vi "oldVisionToGame.vi"(4 "VSS_Ref":T1={"FoulQuadrantVSS"=enum."NO_QUADRANT", "TeamColorVSS"=enum."YELLOW", "HalfVSS"=enum."NO_HALF", "Foul"=enum."FREE_KICK", "timestamp"=0.0}, 5 "Defense stretch":i32=500, 6 "Team/ Side":u16[](array[numeric]), 7 "Defense width":i32=1000, 8 "error in (no error)":errorcluster, 9 "touch":bool, 10 "IA State":T2={"our_robots"=[], "enemy_robots"=[], "balls"=[], "geometry"={"line_width"=0, "field_length"=0, "field_width"=0, "boundary_width"=0, "referee_width"=0, "goal_width"=0, "goal_depth"=0, "goal_wall_width"=0, "center_circle_radius"=0, "defense_radius"=0, "defense_stretch"=0, "free_kick_from_defense_dist"=0, "penalty_spot_from_field_line_dist"=0, "penalty_line_from_spot_dist"=0}, "IA Judge"={"stage"="", "command"="", "our_goalie_id"=0.0, "enemy_goalie_id"=0.0, "command enum"=enum."Halt", "Time"=enum."Azul"}, "Received Timestamp"=timestamp(0 s since 1904-01-01), "Events"={"Touch"=FALSE, "Ball out"=FALSE, "id touch"=0.0, "Ball out of \nVision"=FALSE, "Ball inside \nGoalie area"=FALSE, "Robot not responding"=FALSE, "Robots responding status"=[1.0, 1.0, 1.0, 1.0, 1.0, 1.0], "Enemy Ball \nPossession"=FALSE, "Pass State"=FALSE, "id end of pass"=0.0, "Kick"=FALSE, "Id ini Possession"=0.0, "Ball Possesion"=FALSE, "Id Possesion"=0.0, "Direct Kick"=FALSE, "2nd Strk Ativo"=FALSE}}, 11 "Game in":refnum<class "Game.lvclass">) -> (0 "error out":errorcluster, 3 "Game out":refnum<class "Game.lvclass">)   [LabVIEW 2023, in "Game.lvclass"]
uses:
  Game.lvclass
  Vision_class/Old vision/SSL Detection Frame Simple Estimator Cameras VelCmd Folder/Core/AI Input.ctl
  Vision_class/Old vision/Controls/AI Robot.ctl
  Vision_class/Old vision/Controls/Functions Enum.ctl
  Vision_class/Old vision/Controls/AttackerStates.ctl
  Vision_class/Old vision/Controls/PathDests.ctl
  Vision_class/Old vision/Controls/PathDest.ctl
  Navigation/VSSNavigation/VSSAttackerStates.ctl
  Vision_class/Old vision/SSL Detection Frame Simple Estimator Cameras VelCmd Folder/Core/AI Ball.ctl
  Vision_class/Old vision/SSL Detection Frame Simple Estimator Cameras VelCmd Folder/Core/Field Size.ctl
  Vision_class/Old vision/SSL Detection Frame Simple Estimator Cameras VelCmd Folder/Core/AI Judge.ctl
  Communication_class/Paths/MessageAI_State Folder/Intel/Command Enum.ctl
  Vision_class/Old vision/SSL Detection Frame Simple Estimator Cameras VelCmd Folder/Util/Events/Events.ctl
  Referee_class/VSS_Ref.ctl
  Game.lvclass/Game.ctl
  Write FieldRef.vi
  Write AllyRef.vi
  Write EnemyRef.vi
  Write BallRef.vi
  Write TimeRef.vi
  Write Referee.vi
  Read FieldRef.vi
  Read AllyRef.vi
  Read EnemyRef.vi
  Read BallRef.vi
  Read Referee.vi
  Field_class/Field.lvclass
  Ally_class/Ally.lvclass
  Enemy_class/Enemy.lvclass
  Ball_class/Ball.lvclass
  Referee_class/Referee.lvclass
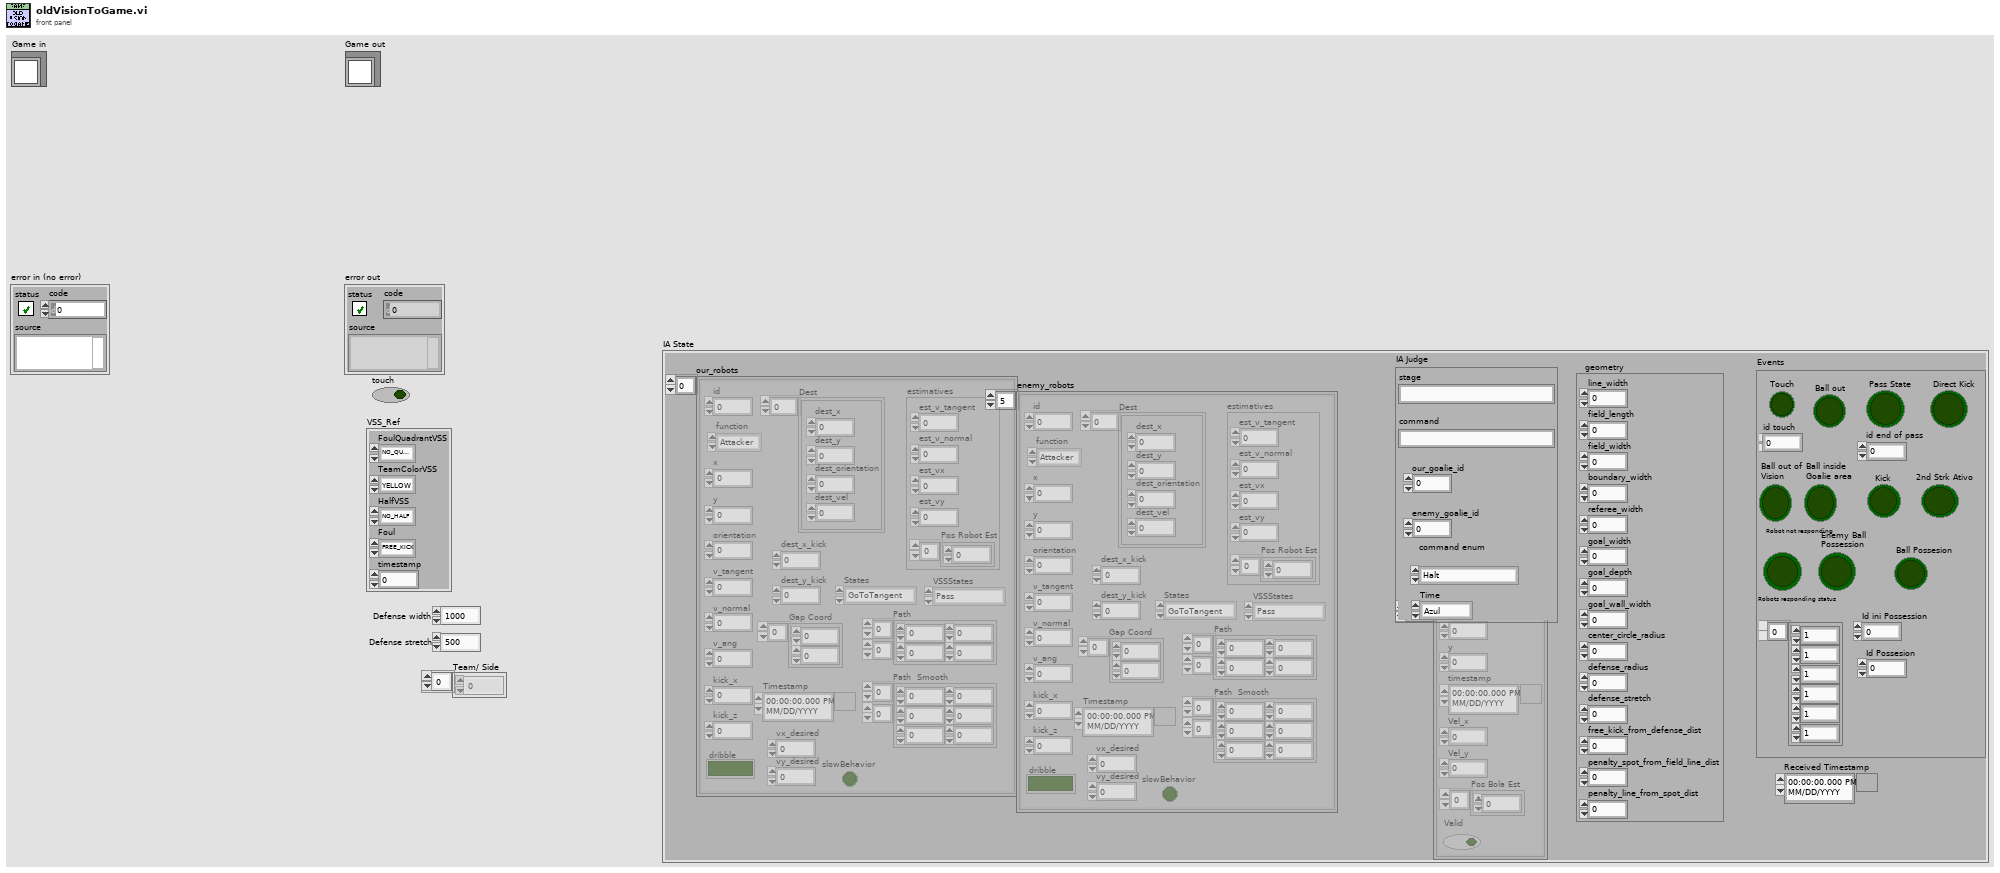
[diagram p1: front panel]
types:
  T1 = typedef "VSS_Ref.ctl" = cluster{"FoulQuadrantVSS":enum16{"NO_QUADRANT", "QUADRANT_1", "QUADRANT_2", "QUADRANT_3", "QUADRANT_4"}, "TeamColorVSS":enum16{"BLUE", "YELLOW", "NONE"}, "HalfVSS":enum16{"NO_HALF", "FIRST_HALF", "SECOND_HALF", "OVERTIME_FIRST_HALF", "OVERTIME_SECOND_HALF", "PENALTY_SHOOTOUS"}, "Foul":enum16{"FREE_KICK", "PENALTY_KICK", "GOAL_KICK", "FREE_BALL", "KICKOFF", "STOP", "GAME_ON", "HALT"}, "timestamp":dbl}
  T2 = typedef "AI Input.ctl" = cluster{"our_robots":T3[], "enemy_robots":T3[], "balls":T9[], "geometry":T10, "IA Judge":T11, "Received Timestamp":timestamp, "Events":T13}
  T3 = typedef "AI Robot.ctl" = cluster{"id":u32, "function":T4, "x":dbl, "y":dbl, "orientation":dbl, "v_tangent":dbl, "v_normal":dbl, "v_ang":dbl, "kick_x":dbl, "kick_z":dbl, "dribble":bool, "Timestamp":timestamp, "estimatives":cluster{"est_v_tangent":dbl, "est_v_normal":dbl, "est_vx":dbl, "est_vy":dbl, "Pos Robot Est":dbl[]}, "dest_x_kick":dbl, "dest_y_kick":dbl, "Gap Coord":dbl[], "States":T5, "Path ":dbl[][], "Path  Smooth":dbl[][], "Dest":T6, "vx_desired":dbl, "vy_desired":dbl, "slowBehavior":bool, "VSSStates":T8}
  T4 = typedef "Functions Enum.ctl" = enum16{"2nd Striker", "Attacker", "Goalie", "Defender", "Striker", "Goto 0", "Dummy", "Kicker", "ZigZag 0", "ZigZag 1", "ZigZag 2", "ZigZag 3", "ZigZag 4", "ZigZag 5", "ZigZag 6", "ZigZag 7", "ZigZag 8", ""}
  T5 = typedef "AttackerStates.ctl" = enum16{"Pass", "GoToTangent", "BallGetting", "GoToKick", ""}
  T6 = typedef "PathDests.ctl" = T7[]
  T7 = typedef "PathDest.ctl" = cluster{"dest_x":dbl, "dest_y":dbl, "dest_orientation":dbl, "dest_vel":dbl}
  T8 = typedef "VSSAttackerStates.ctl" = enum16{"Pass", "GoToTangent", "BallGetting", "GoToKick", "Rotate anti-clockwise", "Rotate Clockwise", ""}
  T9 = typedef "AI Ball.ctl" = cluster{"x":dbl, "y":dbl, "timestamp":timestamp, "Vel_x":dbl, "Vel_y":dbl, "Pos Bola Est":dbl[], "Valid":bool}
  T10 = typedef "Field Size.ctl" = cluster{"line_width":u32, "field_length":u32, "field_width":u32, "boundary_width":u32, "referee_width":u32, "goal_width":u32, "goal_depth":u32, "goal_wall_width":u32, "center_circle_radius":u32, "defense_radius":u32, "defense_stretch":u32, "free_kick_from_defense_dist":u32, "penalty_spot_from_field_line_dist":u32, "penalty_line_from_spot_dist":u32}
  T11 = typedef "AI Judge.ctl" = cluster{"stage":string, "command":string, "our_goalie_id":dbl, "enemy_goalie_id":dbl, "command enum":T12, "Time":enum16{"Azul", "Amarelo"}}
  T12 = typedef "Command Enum.ctl" = enum16{"Halt", "Stop", "Force Start", "PKA Normal Start", "Prepare Kickoff Ally", "PKE Normal Start", "Prepare Kickoff Enemy", "Prepare Penalty Ally", "PPA Normal Start", "Prepare Penalty Enemy", "PPE Normal Start", "Direct Free Enemy", "Direct Free Ally", "Indirect Free Enemy", "Indirect Free Ally", "Timeout Enemy", "Timeout Ally", "Goal Enemy", "Goal Ally", "Ball Placement Enemy", "Ball Placement Ally", "Normal Half Time", "Extra Time Break", "Extra Half Time", "None", "Post Game"}
  T13 = typedef "Events.ctl" = cluster{"Touch":bool, "Ball out":bool, "id touch":dbl, "Ball out of \nVision":bool, "Ball inside \nGoalie area":bool, "Robot not responding":bool, "Robots responding status":dbl[], "Enemy Ball \nPossession":bool, "Pass State":bool, "id end of pass":dbl, "Kick":bool, "Id ini Possession":dbl, "Ball Possesion":bool, "Id Possesion":dbl, "Direct Kick":bool, "2nd Strk Ativo":bool}
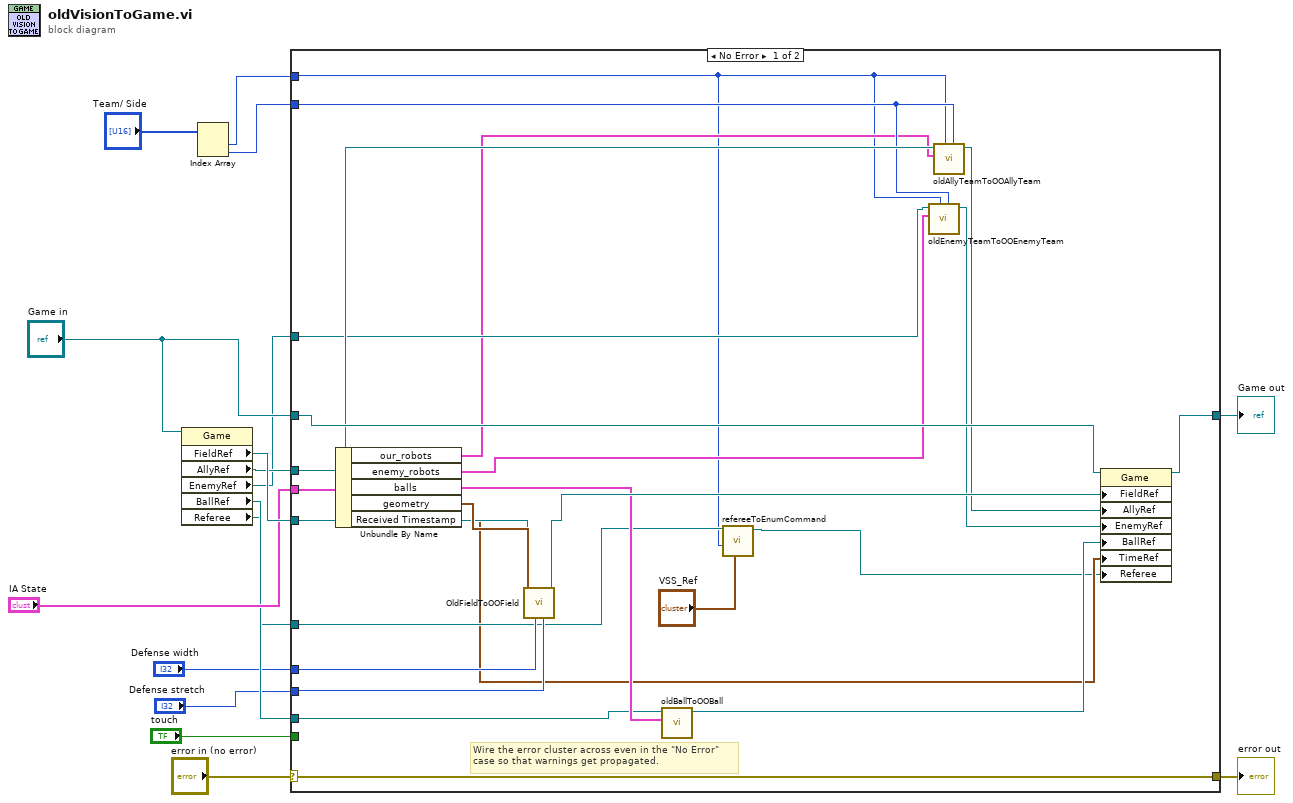
[diagram p0: block diagram]
diagram:
  n1 = property class="Game"(reference="Game in") -> ("FieldRef"=w12:refnum<class "Field.lvclass">, "AllyRef"=w11:refnum<class "Ally.lvclass">, "EnemyRef"=w10:refnum<class "Enemy.lvclass">, "BallRef"=w5:refnum<class "Ball.lvclass">, "Referee"=w2:refnum<class "Referee.lvclass">)  [unwired: 1 in, 2 out]
  n2 = Index Array(array="Team/ Side") -> (element #1=w8:u16, element #2=w7:u16)  [unwired: 2 in]
  n3 = case shown="No Error" "error in (no error)" {
    selector: "error in (no error)" -> [w40 w42]
    tunnel: [w40 w42] -> w15
    tunnel: [w36 w41] -> w14
    tunnel: "Game in" -> [w35 w41]
    tunnel: "IA State" -> [w21 _]
    tunnel: w12 -> [w38 _]
    tunnel: w7 -> [w29 _]
    tunnel: w11 -> [w33 _]
    tunnel: w10 -> [w32 _]
    tunnel: w8 -> [w17 _]
    tunnel: w5 -> [w25 _]
    tunnel: "Defense width" -> [w24 _]
    tunnel: "Defense stretch" -> [w23 _]
    tunnel: w2 -> [w22 _]
    tunnel: "touch" -> [_ _]
    frame No Error {
      # "Wire the error cluster across even in the \"No Error\"\ncase so that warnings get propagated."
      n4 = Unbundle By Name(w21) -> ("our_robots"=w26:T3[], "enemy_robots"=w28:T3[], "balls"=w27:T9[], "geometry"=w39:T10, "Received Timestamp"=w20:timestamp)
      n5 = call "OldFieldToOOField.vi"("Defense stretch"=w23, "Defense width"=w24, "geometry"=w39, "Field in"=w38) -> ("Field out"=w37:refnum<class "Field.lvclass">)  [unwired: 6 in, 1 out]
      n6 = call "oldBallToOOBall.vi"("balls"=w27, "Ball in"=w25) -> ("Ball out"=w30:refnum<class "Ball.lvclass">)  [unwired: 8 in, 1 out]
      n7 = call "refereeToEnumCommand.vi"("VSS_Ref"="VSS_Ref", "team"=w17, "Referee in"=w22) -> ("Referee out"=w18:refnum<class "Referee.lvclass">)  [unwired: 7 in, 1 out]
      n8 = call "oldEnemyTeamToOOEnemyTeam.vi"("Side"=w29, "Team"=w17, "enemy_robots"=w28, "Enemy in"=w32) -> ("Enemy out"=w31:refnum<class "Enemy.lvclass">)  [unwired: 6 in, 1 out]
      n9 = call "oldAllyTeamToOOAllyTeam.vi"("Side"=w29, "Team"=w17, "our_robots"=w26, "Ally in"=w33) -> ("Ally out"=w34:refnum<class "Ally.lvclass">)  [unwired: 6 in, 1 out]
      n10 = property class="Game"(reference=w35, "FieldRef"=w37, "AllyRef"=w34, "EnemyRef"=w31, "BallRef"=w30, "TimeRef"=w20, "Referee"=w18) -> (reference out=w36:refnum<class "Game.lvclass">)  [unwired: 1 in, 1 out]
    }
    frame Error {
    }
  }
  "error out" <- w15
  "Game out" <- w14
